vi "digitalstyrsignal.vi"() -> ()   [LabVIEW 2012]
uses:
  <vilib>/DAQmx/write.llb/DAQmx Write (Digital 1D Bool NChan 1Samp 1Line).vi
  <vilib>/DAQmx/miscellaneous.llb/DAQmx Fill In Error Info.vi
panel:
  in  "Strömbrytare":bool
  in  "16":bool
  in  "13":bool
  in  "14":bool
  in  "15":bool
  in  "10":bool
  in  "11":bool
  in  "12":bool
  in  "7":bool
  in  "8":bool
  in  "9":bool
  in  "4":bool
  in  "5":bool
  in  "6":bool
  in  "1":bool
  in  "2":bool
  in  "3":bool
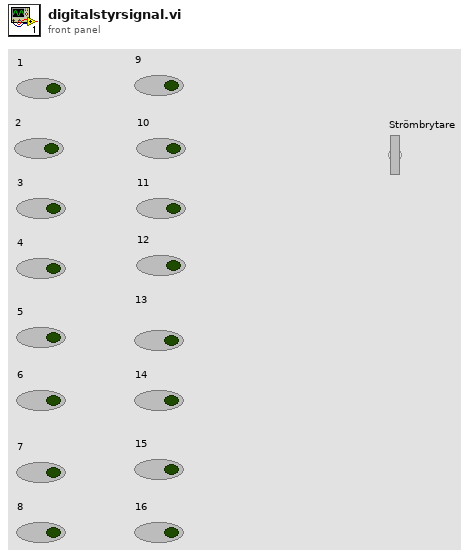
[diagram p1: front panel]
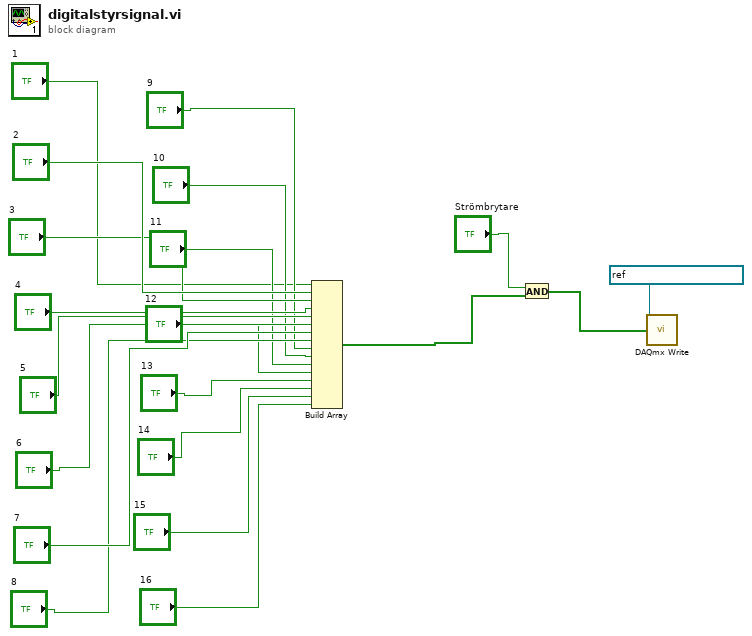
[diagram p0: block diagram]
diagram:
  n1 = Build Array("1", "2", "3", "4", "5", "6", "7", "8", "9", "10", "11", "12", "13", "14", "15", "16") -> (w4:bool[])
  n2 = And(x="Strömbrytare", y=w4) -> (x .and. y?=w3:bool[])
  n3 = call-poly <vilib>:"DAQmx Write.vi"("task/channels in"=refnum<k21> "MyDigitalOutTask_2", "data"=w3) -> ()  [unwired: 11 in, 3 out]
